vi "1_OnInterrupts_Raw_Fast.vi"() -> ()   [LabVIEW 2020]
uses:
  <vilib>/Instr/_visa.llb/VISA Configure Serial Port (Instr).vi
  <vilib>/express/express analysis/Spectral/Block/exnSpectralBlock spectral measurements RMS poly.vi
  <vilib>/express/express analysis/Spectral/Block/exnSpectralBlock spectral measurements RMS WFM.vi
  <vilib>/express/express analysis/Spectral/XNode/ExpressSpectralMeasurementsBlockNode.xnode
panel:
  in  "stop":bool
  in  "Tab Control":enum32{"Main", "Freq", "Service"}(tab)
  out "Measurement":u8[](graph)
  out "Spectrum":cluster{"f0":dbl, "df":dbl, "magnitude":dbl[]}(graph)
  out "error out":errorcluster
  in  "VISA resource name":refnum<visa-resource-name>="COM7"
  out "answer":string="673 \n\r"
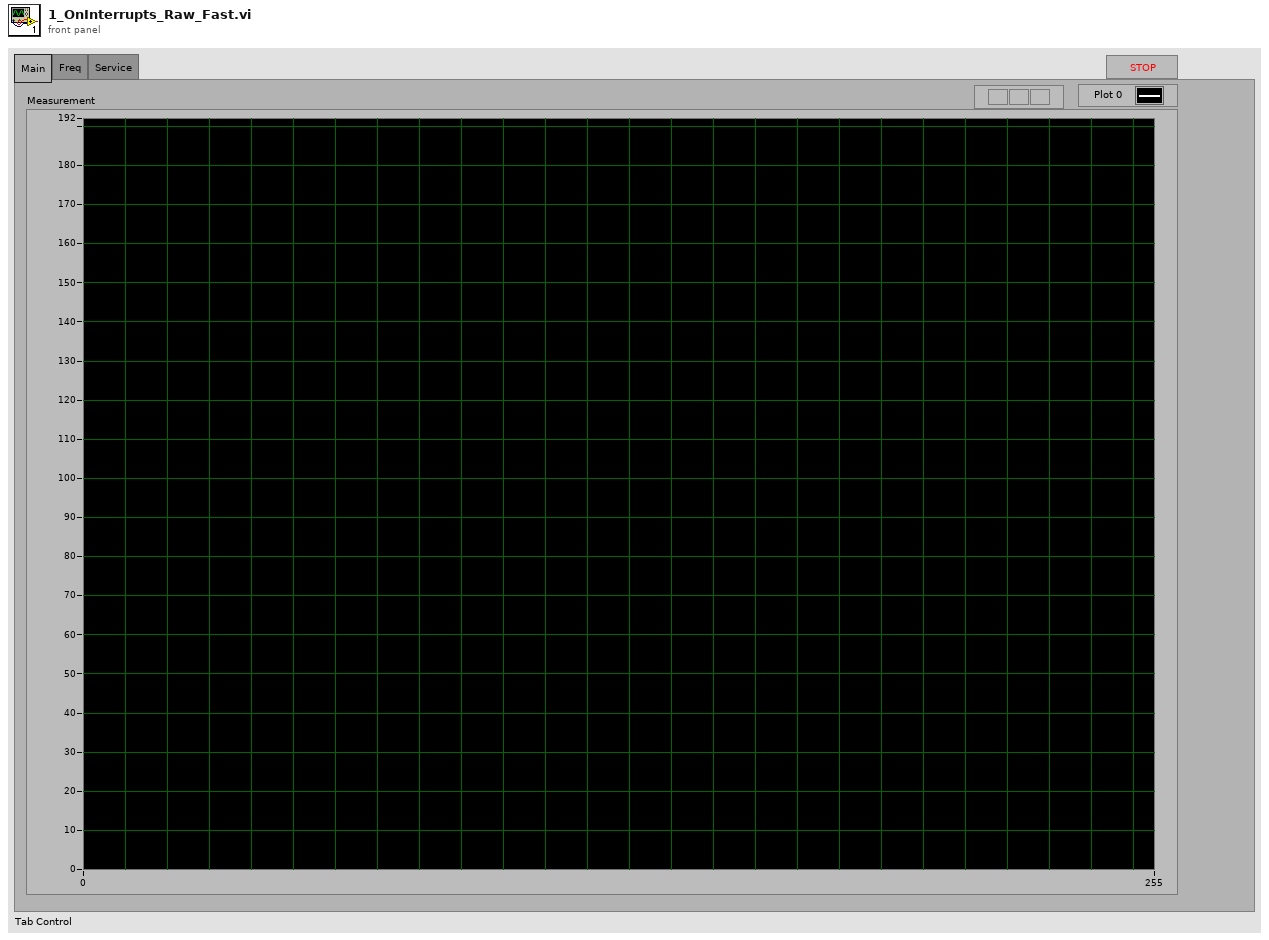
[diagram p1: front panel]
types:
  T1 = cluster{"averaging mode":u16, "weighting mode":u16, "number of averages":u32}
  T2 = cluster{"dB On (F)":bool, "unwrap phase (F)":bool, "convert to degree (F)":bool}
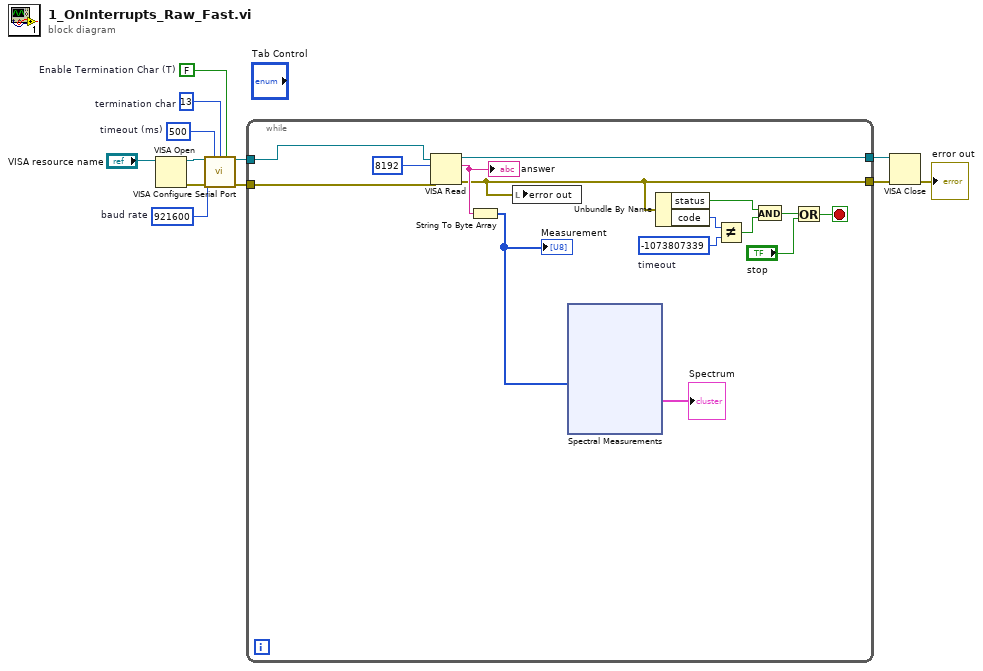
[diagram p0: block diagram]
diagram:
  w1 = u32 921600  # baud rate
  w2 = u32 500  # timeout (ms)
  w8 = FALSE  # Enable Termination Char (T)
  w9 = u8 13  # termination char
  n1 = VISA Open(VISA resource name="VISA resource name") -> (VISA resource name=w11:refnum<visa-resource-name>, error out=w12:errorcluster)  [unwired: 4 in]
  n2 = call-poly "VISA Configure Serial Port"("VISA resource name"=w11, "timeout (10sec)"=w2, "termination char\n(0xA = '\\n' = LF)"=w9, "Enable Termination\nChar (T)"=w8, "baud rate (9600)"=w1, "error in (no error)"=w12) -> ("VISA resource name out"=w5:refnum<visa-resource-name>, "error out"=w4:errorcluster)  [unwired: 8 in]
  n3 = while {
    tunnel: w5 -> [w26]
    tunnel: [w27] -> w7
    tunnel: w4 -> [w15]
    tunnel: [w23] -> w6
    stop <- w17 stop-if-true
    w21 = -1073807339  # timeout
    n4 = VISA Read(VISA resource name=w26, byte count=u32 8192, error in (no error)=w15) -> (VISA resource name out=w27:refnum<visa-resource-name>, read buffer=w24:string, error out=w23:errorcluster)  [unwired: 1 out]
    "answer" <- w24
    n5 = String To Byte Array(string=w24) -> (unsigned byte array=w13:u8[])
    "Measurement" <- w13
    n6 = local write "error out"(w23) -> ()
    n7 = xnode "Spectral Measurements"("Signals"=w13) -> ("FFT - (RMS)"=→"Spectrum":cluster{"f0":dbl, "df":dbl, "magnitude":dbl[]})  [unwired: 1 in, 2 out]
    n8 = Unbundle By Name(w23) -> ("status"=w19:bool, "code"=w22:i32)
    n9 = Not Equal?(x=w22, y=w21) -> (x != y?=w20:bool)
    n10 = And(x=w19, y=w20) -> (x .and. y?=w18:bool)
    n11 = Or(x=w18, y="stop") -> (x .or. y?=w17:bool)
  }
  n12 = VISA Close(VISA resource name=w7, error in (no error)=w6) -> (error out=→"error out":errorcluster)
